vi "Ballard 429 - Initialize - Get Tx Messages Handles.vi"(8 "error in (no error)":errorcluster, 10 "channel handles[]":u64[](array[numeric]), 11 "Tx Config in":T1[](array[typedef]) {"Labels Settings"."Label Timestamp Channel Data Reference" format="%.0x"; "Labels Settings"."Label Disable/Trigger Channel Reference" format="%.0x"; "Labels Settings"."Word"."Param Setting"."Item Refs" format="%.0x"; "Labels Settings"."Word"."Param Setting"."Num Bits" min=1 max=32; "Labels Settings"."Word"."Param Setting"."Start Bit" min=8 max=31; "Labels Settings"."Label" format="%.0o"}) -> (0 "error out":errorcluster, 3 "Tx Config out":T1[](array[typedef]) {"Labels Settings"."Label Timestamp Channel Data Reference" format="%.0x"; "Labels Settings"."Label Disable/Trigger Channel Reference" format="%.0x"; "Labels Settings"."Word"."Param Setting"."Item Refs" format="%.0x"; "Labels Settings"."Word"."Param Setting"."Num Bits" min=1 max=32; "Labels Settings"."Word"."Param Setting"."Start Bit" min=8 max=31; "Labels Settings"."Label" format="%.0o"})   [LabVIEW 2020, in "Ballard Arinc-429 Engine.lvlib"]
doc: "For all Tx Channels, we fetch Channel Handle and Message Handle (if Scheduled Labels)."
uses:
  Ballard Arinc-429 Engine.lvlib
  Shared/Controls and Global/RT HW Channel.ctl
  Shared/Controls and Global/RT Label Settings.ctl
  Shared/Controls and Global/Label.ctl
  Shared/Controls and Global/transferPeriod.ctl
  Shared/Controls and Global/RT Word Settings.ctl
  Shared/Controls and Global/RT Param Setting.ctl
  Shared/Controls and Global/Start Bit.ctl
  Shared/Controls and Global/Number of Bits.ctl
  <vilib>/NI VeriStand/Custom Device API/Block Data Reference.ctl
  <vilib>/NI VeriStand/Custom Device API/Data Reference.ctl
  <vilib>/NI VeriStand/Custom Device API/Custom Device Item Ref.ctl
  Shared/Controls and Global/TransferType.ctl
  <instrlib>/BTI429Lib/BTI429LV.lvlib
  Shared/Ballard Arinc-429 Shared.lvlib
  <vilib>/NI VeriStand/Custom Device API/Custom Device API.lvlib
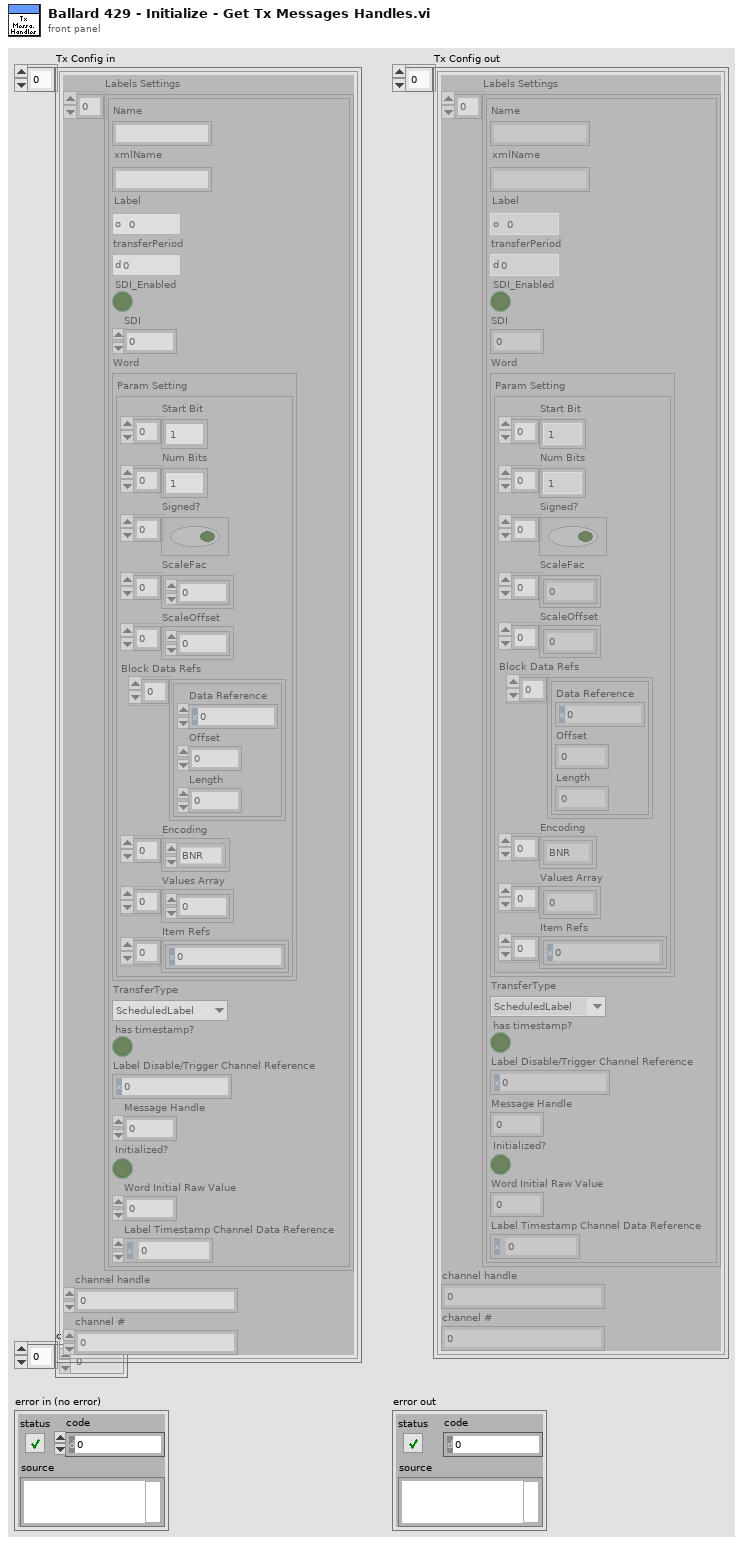
[diagram p1: front panel]
types:
  T1 = typedef "Ballard Arinc-429 Shared.lvlib/RT HW Channel.ctl" = cluster{"Labels Settings":T2[], "channel handle":u64, "channel #":u16}
  T2 = typedef "Ballard Arinc-429 Shared.lvlib/RT Label Settings.ctl" = cluster{"Name":string, "xmlName":string, "Label":T3, "transferPeriod":T4, "SDI_Enabled":bool, "SDI":u8, "Word":T5, "TransferType":T12, "has timestamp?":bool, "Label Disable/Trigger Channel Reference":T11, "Message Handle":u64, "Initialized?":bool, "Word Initial Raw Value":u32, "Label Timestamp Channel Data Reference":T10}
  T3 = typedef "Ballard Arinc-429 Shared.lvlib/Label.ctl" = u8
  T4 = typedef "Ballard Arinc-429 Shared.lvlib/transferPeriod.ctl" = u32
  T5 = typedef "Ballard Arinc-429 Shared.lvlib/RT Word Settings.ctl" = cluster{"Param Setting":T6}
  T6 = typedef "Ballard Arinc-429 Shared.lvlib/RT Param Setting.ctl" = cluster{"Start Bit":T7[], "Num Bits":T8[], "Signed?":bool[], "ScaleFac":dbl[], "ScaleOffset":dbl[], "Block Data Refs":T9[], "Encoding":enum16{"BNR", "BCD", "Discrete"}[], "Values Array":dbl[], "Item Refs":T11[]}
  T7 = typedef "Ballard Arinc-429 Shared.lvlib/Start Bit.ctl" = i32
  T8 = typedef "Ballard Arinc-429 Shared.lvlib/Number of Bits.ctl" = i32
  T9 = typedef "Custom Device API.lvlib/Block Data Reference.ctl" = cluster{"Data Reference":T10, "Offset":u64, "Length":u64}
  T10 = typedef "Custom Device API.lvlib/Data Reference.ctl" = i32
  T11 = typedef "Custom Device API.lvlib/Custom Device Item Ref.ctl" = u64
  T12 = typedef "Ballard Arinc-429 Shared.lvlib/TransferType.ctl" = enum16{"ScheduledLabel", "Acyclic", "Block", "Strobe"}
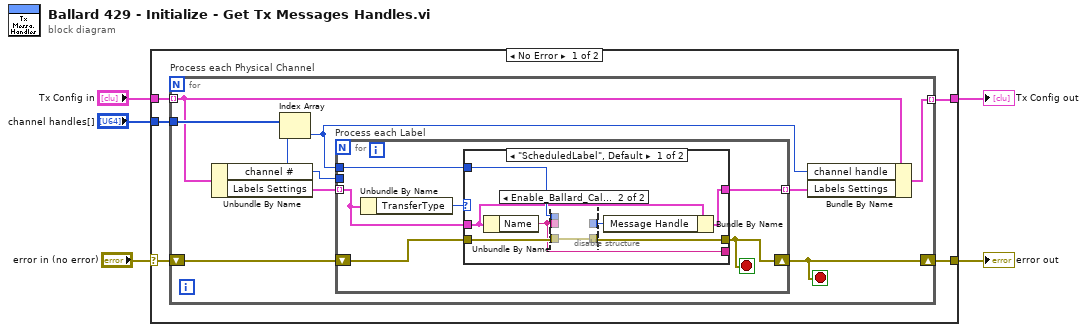
[diagram p0: block diagram]
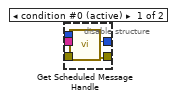
[diagram p2: hidden frame]
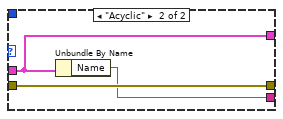
[diagram p3: hidden frame]
diagram:
  n1 = case shown="No Error" "error in (no error)" {
    selector: "error in (no error)" -> [w6 w42]
    tunnel: "channel handles[]" -> [w10 _]
    tunnel: "Tx Config in" -> [w9 w43]
    tunnel: [w8 w43] -> w3
    tunnel: [w7 w42] -> w5
    frame No Error {
      n2 = for "Process each Physical Channel" {
        tunnel: w9 -> [w16] mode=indexing
        tunnel: w10 -> [w19]
        tunnel: [w15] -> w8 mode=indexing
        shift-right: [w12] -> w7
        shift-left: w6 -> [w18]
        stop <- w12 stop-if-true
        n3 = Unbundle By Name(w16) -> ("channel #"=w13:u16, "Labels Settings"=w17:T2[])
        n4 = Index Array(array=w19, index=w13) -> (element=w11:u64)
        n5 = for "Process each Label" {
          tunnel: w17 -> [w22] mode=indexing
          tunnel: w11 -> [w23]
          tunnel: [w24] -> w14 mode=indexing
          shift-right: [w20] -> w12
          shift-left: w18 -> [w25]
          tunnel: w13 -> [_]
          stop <- w20 stop-if-true
          n6 = Unbundle By Name(w22) -> ("TransferType"=w21:T12)
          n7 = case shown="\"ScheduledLabel\", Default" w21 {
            tunnel: w25 -> [w32 w41]
            tunnel: [w31 w40] -> w24
            tunnel: w23 -> [w29 _]
            tunnel: [w28 w41] -> w20
            tunnel: w22 -> [w27 w40]
            tunnel: [w26 w39] -> _
            frame "ScheduledLabel", Default {
              n8 = Unbundle By Name(w27) -> ("Name"=w26:string)
              n9 = disable-structure shown="Enable_Ballard_Calls==False" {
                disable-tunnel: w32 -> [w37 w38]
                disable-tunnel: [w36 _] -> w30
                disable-tunnel: w29 -> [w35 _]
                disable-tunnel: [w34 w38] -> w28
                disable-tunnel: w26 -> [w33 _]
                frame condition #0 (active) {
                  n10 = call <instrlib>:"Get Scheduled Message Handle.vi"("error in (no error)"=w37, "message name"=w33, "channel handle in"=w35) -> ("error out"=w34:errorcluster, "message handle out"=w36:u64)  [unwired: 6 in, 1 out]
                }
                frame condition #1 {
                }
              }
              n11 = Bundle By Name(cluster=w27, "Message Handle"=w30) -> (w31:T2)
            }
            frame "Acyclic" {
              n12 = Unbundle By Name(w40) -> ("Name"=w39:string)
            }
          }
        }
        n13 = Bundle By Name(cluster=w16, "channel handle"=w11, "Labels Settings"=w14) -> (w15:T1)
      }
    }
    frame Error {
    }
  }
  "error out" <- w5
  "Tx Config out" <- w3
